vi "Intake Compression Immediate_wrapper.vi"(7 "Description":string, 8 "Command Info In":T1, 11 "Intake Roller Speed":dbl) -> (0 "Command Info Out":T1)   [LabVIEW 2025]
uses:
  <vilib>/Rock Robotics/WPI/Framework/Completion Status.ctl
  <vilib>/Rock Robotics/WPI/Framework/Completion Notifier.ctl
  <vilib>/Rock Robotics/WPI/Framework/Command Status Info.ctl
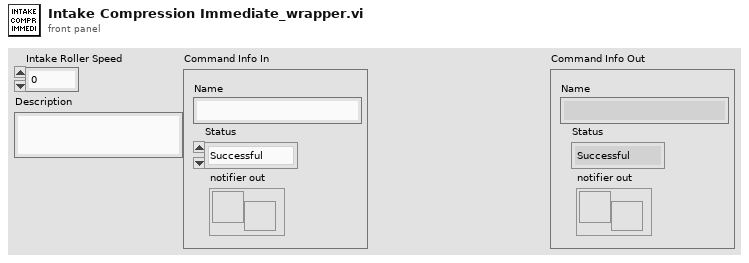
[diagram p1: front panel]
types:
  T1 = typedef "Command Status Info.ctl" = cluster{"Name":string, "Status":T2, "notifier out":T3}
  T2 = typedef "Completion Status.ctl" = enum16{"Successful", "Aborted", "Incomplete"}
  T3 = typedef "Completion Notifier.ctl" = refnum<notifier>
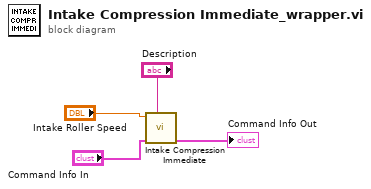
[diagram p0: block diagram]
diagram:
  n1 = call "Intake Compression Immediate.vi"("Description"="Description", "Command Info In"="Command Info In", "Intake Roller Speed"="Intake Roller Speed") -> ("Command Info Out"=→"Command Info Out":T1)  [unwired: 8 in]
